vi "Data Receiver and Reader.vi"() -> ()   [LabVIEW 2016]
uses:
  <vilib>/Utility/file.llb/Read Delimited Spreadsheet (DBL).vi
panel:
  in  "File Path":path=path "C:/Users/Samak/Desktop/LABVIEW Training/Numeric Data Transfer from LabVIEW to-fro File with File IO/Random Data"
  out "Data (All Rows)":dbl[][](array[numeric])
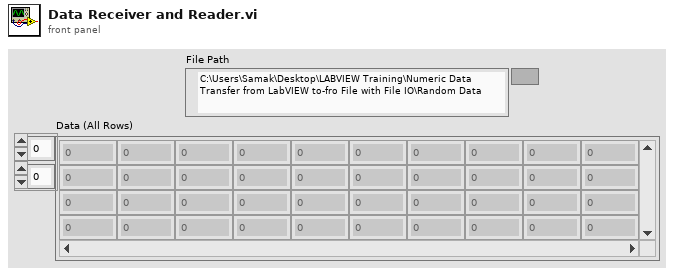
[diagram p1: front panel]
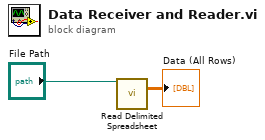
[diagram p0: block diagram]
diagram:
  n1 = call-poly <vilib>:"Read Delimited Spreadsheet.vi"("file path (dialog if empty)"="File Path") -> ("all rows"=→"Data (All Rows)":dbl[][])  [unwired: 9 in, 5 out]
